vi "Write Direccion.vi"(8 "error in (no error)":errorcluster, 10 "Direccion":path, 11 "Logging_txt in":refnum<class "Logging_txt.lvclass">) -> (0 "error out":errorcluster, 3 "Logging_txt out":refnum<class "Logging_txt.lvclass">)   [LabVIEW 2019, in "Logging_txt.lvlib" / "Logging_txt.lvclass"]
uses:
  Logging_txt.lvclass
  Logging_txt.lvclass/Logging_txt.ctl
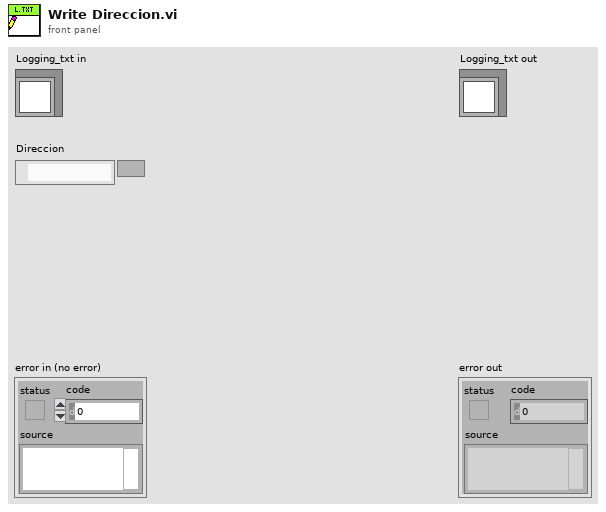
[diagram p1: front panel]
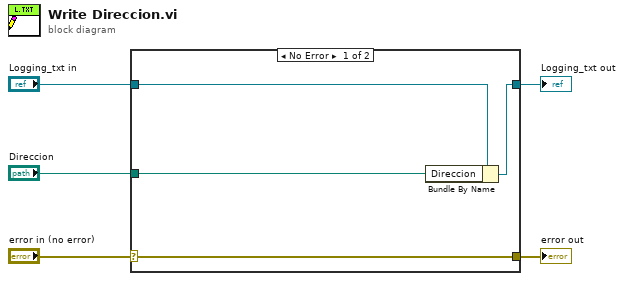
[diagram p0: block diagram]
diagram:
  n1 = case shown="No Error" "error in (no error)" {
    selector: "error in (no error)" -> [w9 w10]
    tunnel: [w9 w10] -> w4
    tunnel: [w7 w11] -> w2
    tunnel: "Logging_txt in" -> [w8 w11]
    tunnel: "Direccion" -> [w6 _]
    frame No Error {
      n2 = Bundle By Name(cluster=w8, "Direccion"=w6) -> (w7:refnum<class "Logging_txt.lvclass">)
    }
    frame Error {
    }
  }
  "error out" <- w4
  "Logging_txt out" <- w2
